vi "Connect Error Controls to Nodes.vi"(4 "error case tunnels in":cluster{"in":refnum<vi>, "out":refnum<vi>}, 6 "error terminals in":cluster{"in":refnum<vi>, "out":refnum<vi>}, 8 "error in (no error)":errorcluster, 10 "case structure in":refnum<vi>, 11 "VI in":refnum<vi>) -> (0 "error out":errorcluster, 2 "case structure out":refnum<vi>, 3 "VI out":refnum<vi>)   [LabVIEW 2017]
uses:
  <vilib>/Utility/miscctls.llb/LVDeltaXY32Cluster.ctl
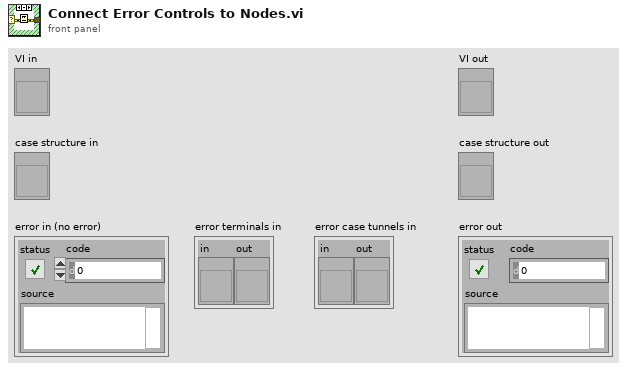
[diagram p1: front panel]
types:
  T1 = typedef "LVDeltaXY32Cluster.ctl" = cluster{"X":i32, "Y":i32}
  T2 = typedef "LVPositionTypeDef.ctl" = cluster{"Left":i32, "Top":i32}
  T3 = typedef "LVRectTypeDef.ctl" = cluster{"Left":i16, "Top":i16, "Right":i16, "Bottom":i16}
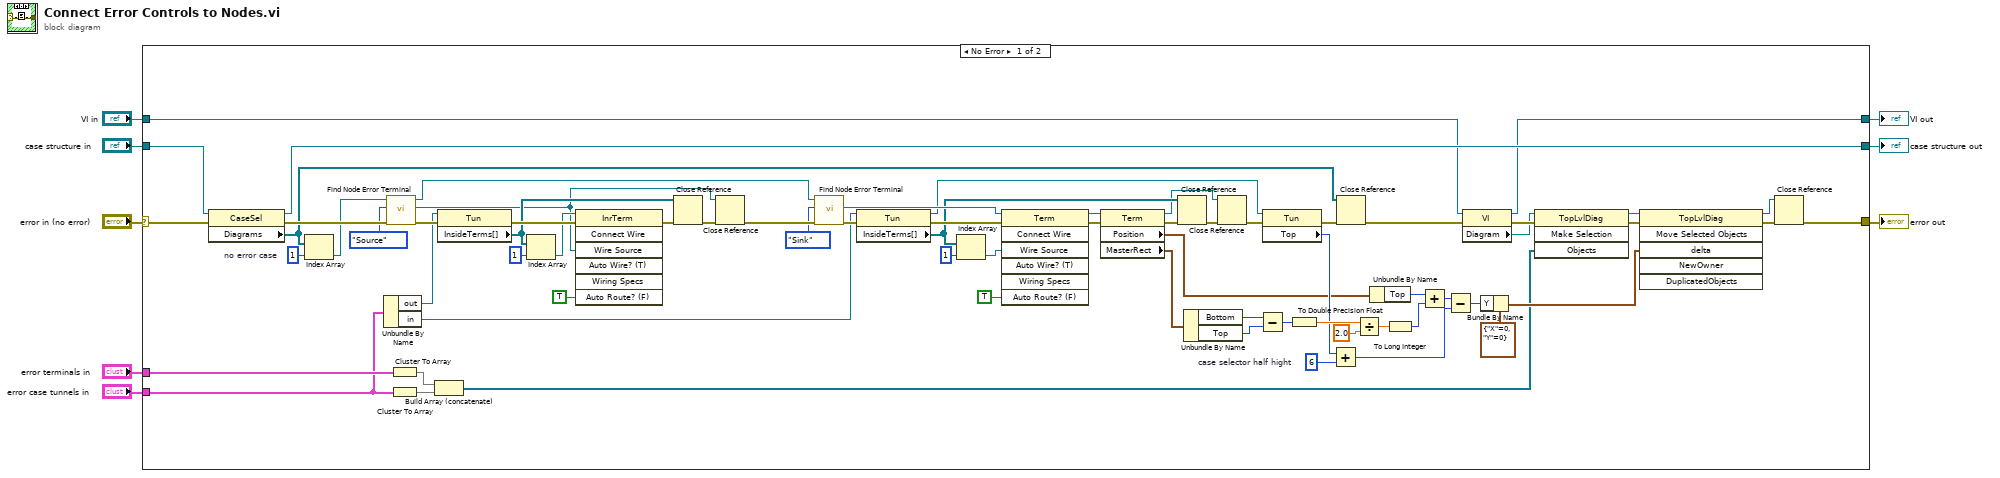
[diagram p0: block diagram]
diagram:
  n1 = case shown="No Error" "error in (no error)" {
    selector: "error in (no error)" -> [w10 w80]
    tunnel: [w73 w79] -> w8
    tunnel: "case structure in" -> [w45 w79]
    tunnel: "error terminals in" -> [w38 _]
    tunnel: "error case tunnels in" -> [w36 _]
    tunnel: "VI in" -> [w32 w78]
    tunnel: [w31 w78] -> w3
    tunnel: [w29 w80] -> w2
    frame No Error {
      w65 = 6  # case selector half hight
      w39 = 1  # no error case
      n2 = property class="CaseSel"(reference=w45, error in=w10) -> (reference out=w73:refnum<vi>, error out=w44:errorcluster, "Diagrams"=w11:refnum<vi>[])
      n3 = Index Array(array=w11, index=w39) -> (element=w42:refnum<vi>)
      n4 = Unbundle By Name(w36) -> ("out"=w13:refnum<vi>, "in"=w55:refnum<vi>)
      n5 = call "Find Node Error Terminal.vi"("error in (no erros)"=w44, "source/sink"=enum16{"Source", "Sink"}."Source", "diagram in"=w42) -> ("error out"=w74:errorcluster, "error terminal"=w24:refnum<vi>, "diagram out"=w43:refnum<vi>)  [unwired: 6 in]
      n6 = Cluster To Array(cluster=w38) -> (array=w37:refnum<vi>[])
      n7 = Cluster To Array(cluster=w36) -> (array=w35:refnum<vi>[])
      n8 = Build Array (concatenate)(w37, w35) -> (w34:refnum<vi>[])
      n9 = property class="Tun"(reference=w13, error in=w74) -> (error out=w75:errorcluster, "InsideTerms[]"=w25:refnum<vi>[])  [unwired: 1 out]
      n10 = Index Array(array=w25, index=1) -> (element=w26:refnum<vi>)
      n11 = invoke class="InrTerm" method="Connect Wire"(reference=w26, error in=w75, "Wire Source"=w24, "Auto Route? (F)"=TRUE) -> (error out=w48:errorcluster)  [unwired: 3 in, 6 out]
      n12 = Close Reference(reference=w25, error in (no error)=w48) -> (error out=w23:errorcluster)
      n13 = Close Reference(reference=w24, error in (no error)=w23) -> (error out=w76:errorcluster)
      n14 = call "Find Node Error Terminal.vi"("error in (no erros)"=w76, "source/sink"=enum16{"Source", "Sink"}."Sink", "diagram in"=w43) -> ("error out"=w77:errorcluster, "error terminal"=w46:refnum<vi>)  [unwired: 6 in, 1 out]
      n15 = property class="Tun"(reference=w55, error in=w77) -> (reference out=w9:refnum<vi>, error out=w21:errorcluster, "InsideTerms[]"=w16:refnum<vi>[])
      n16 = Index Array(array=w16, index=1) -> (element=w19:refnum<vi>)
      n17 = invoke class="Term" method="Connect Wire"(reference=w46, error in=w21, "Wire Source"=w19, "Auto Route? (F)"=TRUE) -> (reference out=w54:refnum<vi>, error out=w49:errorcluster)  [unwired: 3 in, 5 out]
      n18 = property class="Term"(reference=w54, error in=w49) -> (reference out=w14:refnum<vi>, error out=w70:errorcluster, "Position"=w58:T2, "MasterRect"=w18:T3)
      n19 = Close Reference(reference=w16, error in (no error)=w70) -> (error out=w17:errorcluster)
      n20 = Unbundle By Name(w18) -> ("Bottom"=w52:i16, "Top"=w53:i16)
      n21 = Close Reference(reference=w14, error in (no error)=w17) -> (error out=w15:errorcluster)
      n22 = Subtract(x=w52, y=w53) -> (x-y=w56:i16)
      n23 = property class="Tun"(reference=w9, error in=w15) -> (error out=w71:errorcluster, "Top"=w64:i32)  [unwired: 1 out]
      n24 = To Double Precision Float(number=w56) -> (double precision float=w67:dbl)
      n25 = Add(x=w64, y=w65) -> (x+y=w68:i32)
      n26 = Close Reference(reference=w11, error in (no error)=w71) -> (error out=w12:errorcluster)
      n27 = Divide(x=w67, y=2.0) -> (x/y=w60:dbl)
      n28 = Unbundle By Name(w58) -> ("Top"=w59:i32)
      n29 = To Long Integer(number=w60) -> (32bit integer=w66:i32)
      n30 = Add(x=w59, y=w66) -> (x+y=w69:i32)
      n31 = Subtract(x=w69, y=w68) -> (x-y=w63:i32)
      n32 = property class="VI"(reference=w32, error in=w12) -> (reference out=w31:refnum<vi>, error out=w33:errorcluster, "Diagram"=w30:refnum<vi>)
      n33 = Bundle By Name(cluster=T1 {"X"=0, "Y"=0} ("X/Y Delta"), "Y"=w63) -> (w62:T1)
      n34 = invoke class="TopLvlDiag" method="Make Selection"(reference=w30, error in=w33, "Objects"=w34) -> (reference out=w51:refnum<vi>, error out=w50:errorcluster)  [unwired: 1 in, 2 out]
      n35 = invoke class="TopLvlDiag" method="Move Selected Objects"(reference=w51, error in=w50, "delta"=w62) -> (reference out=w28:refnum<vi>, error out=w72:errorcluster)  [unwired: 3 in, 4 out]
      n36 = Close Reference(reference=w28, error in (no error)=w72) -> (error out=w29:errorcluster)
    }
    frame Error {
    }
  }
  "case structure out" <- w8
  "error out" <- w2
  "VI out" <- w3
